vi "basic-devices.vi"(6 "Juicer":refnum<vi>, 7 "Lickometer":refnum<vi>, 9 "Valve":refnum<vi>, 10 "Speaker":refnum<vi>, 11 "Cluster in":refnum<vi>) -> (3 "User Event out":T1)   [LabVIEW 2015]
uses:
  Rack/Methods/Rack-Init.vi
  Device/Methods/Lickometer-Init.vi
  Rack/Methods/Rack-Config.vi
  Rack/Methods/Rack-Start.vi
  Device/Methods/Speaker-Init.vi
  Device/Methods/Juicer-Init.vi
  Device/Methods/Valve-Init.vi
  Rack/Typedefs/OutputRequest.ctl
  Rack/Typedefs/OutputRequest refnum.ctl
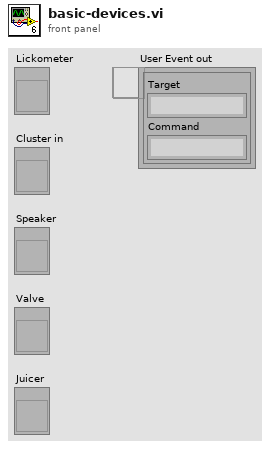
[diagram p1: front panel]
types:
  T1 = typedef "OutputRequest refnum.ctl" = refnum<user-event>
  T2 = typedef "Rack driver configuration cluster.ctl" = cluster{"DigitalInput":T3, "DigitalOutput":T4, "FileOutput":T5, "AnalogOutput":T6, "DataSocketOutput":T7}
  T3 = typedef "DigitalInput-Configuration.ctl" = cluster{"Lines":tag[], "Refresh period (ms)":u32}
  T4 = typedef "DigitalOutput-Configuration.ctl" = cluster{"Output Lines":tag[], "DO timestamp lines":tag[], "Timestamp lines":tag[]}
  T5 = typedef "FileOutput-Configuration.ctl" = cluster{"Logfile path":path}
  T6 = typedef "AnalogOutput-Configuration.ctl" = cluster{"Output Lines":tag[], "AO timestamp lines":tag[]}
  T7 = typedef "DataSocketOutput-Configuration.ctl" = cluster{"DataSocket URL":string}
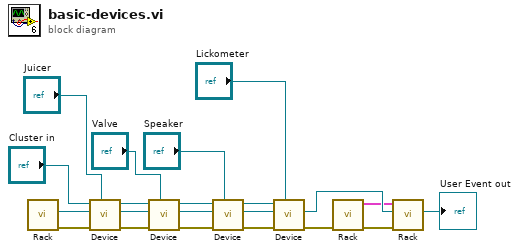
[diagram p0: block diagram]
diagram:
  n1 = call-poly "Rack.vi"() -> ("error out"=w19:errorcluster, "OutputRequest\nevent ref"=w18:T1)  [unwired: 10 in]
  n2 = call-poly "Device.vi"("Device reference"="Juicer", "error in (no error)"=w19, "OutputRequest event ref"=w18, "InputData reference"="Cluster in") -> ("error out"=w16:errorcluster, "OutputRequest (dup)"=w11:T1, "InputData (dup)"=w14:refnum<vi>)  [unwired: 5 in]
  n3 = call-poly "Device.vi"("Device reference"="Valve", "error in (no error)"=w16, "OutputRequest event ref"=w11, "InputData reference"=w14) -> ("error out"=w17:errorcluster, "OutputRequest (dup)"=w12:T1, "InputData (dup)"=w15:refnum<vi>)  [unwired: 5 in]
  n4 = call-poly "Device.vi"("Device reference"="Speaker", "error in (no error)"=w17, "OutputRequest event ref"=w12, "InputData reference"=w15) -> ("error out"=w8:errorcluster, "OutputRequest (dup)"=w7:T1, "InputData (dup)"=w9:refnum<vi>)  [unwired: 5 in]
  n5 = call-poly "Device.vi"("Device reference"="Lickometer", "error in (no error)"=w8, "OutputRequest event ref"=w7, "InputData reference"=w9) -> ("error out"=w1:errorcluster, "OutputRequest (dup)"=w4:T1)  [unwired: 5 in, 1 out]
  n6 = call-poly "Rack.vi"("error in (no error)"=w1) -> ("error out"=w2:errorcluster, "Configuration"=w3:T2)  [unwired: 9 in]
  n7 = call-poly "Rack.vi"("error in (no error)"=w2, "OutputRequest event ref"=w4, "Configuration"=w3) -> ("OutputRequest event ref (dup)"=→"User Event out":T1)  [unwired: 7 in, 1 out]
